vi "Remove Icon Editor Settings.vi"() -> ()   [LabVIEW 2021]
doc: "Clears all Icon Editor keys from the LabVIEW.ini file."
uses:
  <vilib>/Utility/config.llb/NI_LVConfig.lvlib
panel:
  out "error out":errorcluster
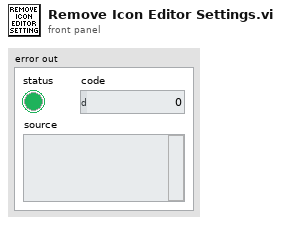
[diagram p1: front panel]
types:
  T1 = typedef "NI_LVConfig.lvlib/Config Data RefNum.ctl" = refnum<k1>
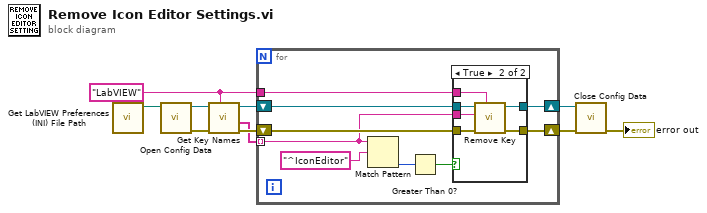
[diagram p0: block diagram]
diagram:
  w1 = "LabVIEW" ("section")
  n1 = call <resource>:"Get LabVIEW Preferences (INI) File Path.vi"() -> ("LabVIEW Preferences (INI) File Path"=w6:path)  [unwired: 11 in]
  n2 = call <vilib>:"Open Config Data.vi"("configuration file path"=w6) -> ("error out"=w10:errorcluster, "refnum"=w5:T1)  [unwired: 8 in, 1 out]
  n3 = call <vilib>:"Get Key Names.vi"("section"=w1, "error in (no error)"=w10, "refnum"=w5) -> ("error out"=w9:errorcluster, "key names"=w2:string[], "refnum out"=w4:T1)  [unwired: 5 in, 1 out]
  n4 = for {
    shift-right: [w16] -> w3
    shift-left: w4 -> [w17]
    shift-right: [w18] -> w8
    shift-left: w9 -> [w19]
    tunnel: w2 -> [w11] mode=indexing
    tunnel: w1 -> [w12]
    n5 = Match Pattern(string=w11, regular expression="^IconEditor") -> (offset past match=w14:i32)  [unwired: 1 in, 3 out]
    n6 = Greater Than 0?(x=w14) -> (x > 0?=w13:bool)
    n7 = case shown="True" w13 {
      tunnel: w17 -> [w20 w25]
      tunnel: [w20 w24] -> w16
      tunnel: w19 -> [w21 w27]
      tunnel: [w21 w26] -> w18
      tunnel: w12 -> [_ w23]
      tunnel: w11 -> [_ w22]
      frame False {
      }
      frame True {
        n8 = call <vilib>:"Remove Key.vi"("section"=w23, "error in (no error)"=w27, "key"=w22, "refnum"=w25) -> ("error out"=w26:errorcluster, "refnum out"=w24:T1)  [unwired: 5 in, 1 out]
      }
    }
  }
  n9 = call <vilib>:"Close Config Data.vi"("error in (no error)"=w8, "refnum"=w3) -> ("error out"=→"error out":errorcluster)  [unwired: 8 in, 1 out]
